vi "DLL Test1.vi"() -> ()   [LabVIEW 2015]
panel:
  out "string":string
  out "Data":string
  out "description":string
  out "VarName":string
  out "initialized array":u8[](array[numeric])
  in  "DLL Path":path
  in  "Load File Path":string="C:\\Users\\Public\\Documents\\National Instruments\\Vision\\Examples\\Images\\Battery\\Image00.jpg"
  in  "Load Template":bool
  in  "coordinate space":bool
  in  "Run":bool
  in  "Enabled/Disabled":bool
  in  "script path":string="C:\\Users\\chenju\\Desktop\\iVision_20160418_Calipter_Coor\\Data\\l"
  in  "stop":bool
  # "<- Run之前要先設定"
  # "<- Run之前要改"
  # "<- Run之前要先設定\n此設定為載入的圖檔"
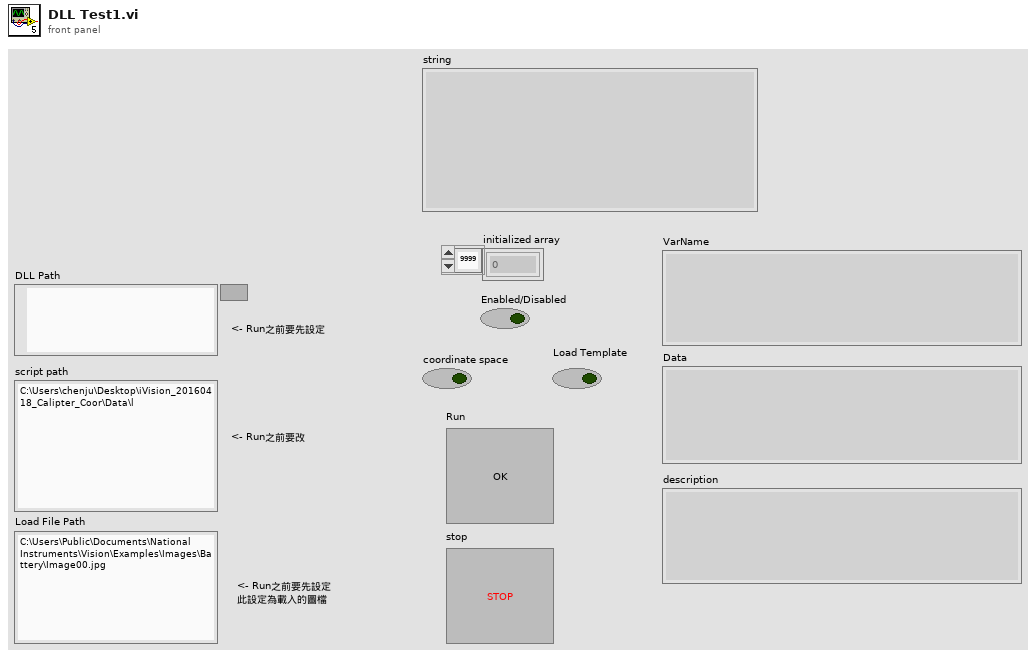
[diagram p1: front panel]
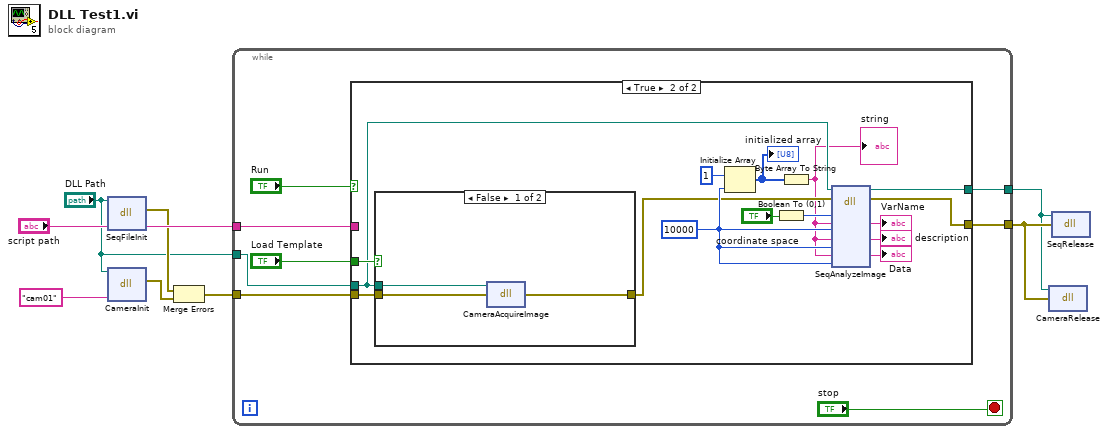
[diagram p0: block diagram]
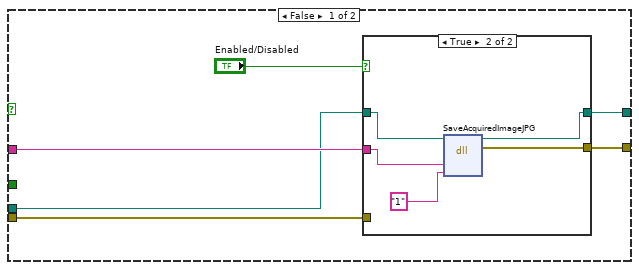
[diagram p2: hidden frame]
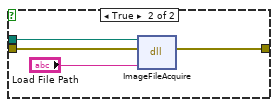
[diagram p4: hidden frame]
diagram:
  n1 = dll-call lib="C:/Users/chenju/Desktop/iVision_20160418_Calipter_Coor/DLL/builds/VisionSeq.dll" fn="SeqFileInit"(path in="DLL Path", "SeqFileInit"="script path") -> (error out=w6:errorcluster, "SeqFileInit"=w7:string)  [unwired: 3 in, 1 out]
  n2 = dll-call lib="C:/Users/chenju/Desktop/iVision_20160418_Calipter_Coor/DLL/builds/VisionSeq.dll" fn="CameraInit"(path in="DLL Path", "CameraInit"="cam01" ("CameraName")) -> (error out=w4:errorcluster)  [unwired: 4 in, 1 out]
  n3 = Merge Errors(w6, w4) -> (w9:errorcluster)
  n4 = while {
    tunnel: w9 -> [w16]
    tunnel: [w15] -> w2
    tunnel: w7 -> [w14]
    tunnel: "DLL Path" -> [w11]
    tunnel: [w10] -> w1
    stop <- "stop" stop-if-true
    n5 = case shown="True" "Run" {
      tunnel: w16 -> [w22 w45]
      tunnel: [w21 w34] -> w15
      tunnel: w14 -> [w20 _]
      tunnel: "Load Template" -> [_ w44]
      tunnel: w11 -> [w18 w33]
      tunnel: [w19 w32] -> w10
      frame False {
        n6 = case shown="True" "Enabled/Disabled" {
          tunnel: w22 -> [w25 _]
          tunnel: [w25 w30] -> w21
          tunnel: w20 -> [_ w27]
          tunnel: [w24 w28] -> w19
          tunnel: w18 -> [w24 w29]
          frame False {
          }
          frame True {
            n7 = dll-call lib="C:/Users/chenju/Desktop/iVision_20160418_Calipter_Coor/DLL/builds/VisionSeq.dll" fn="SaveAcquiredImageJPG"(path in=w29, "Folder Path"=w27, "File Name"="1") -> (path out=w28:path, error out=w30:errorcluster)  [unwired: 5 in]
          }
        }
      }
      frame True {
        w36 = 10000 ("Len")
        n8 = case shown="False" w44 {
          tunnel: w45 -> [w48 w49]
          tunnel: [w47 w50] -> w35
          tunnel: w33 -> [w46 w51]
          frame False {
            n9 = dll-call lib="C:/Users/chenju/Desktop/iVision_20160418_Calipter_Coor/DLL/builds/VisionSeq.dll" fn="CameraAcquireImage"(path in=w46, error in=w48) -> (error out=w47:errorcluster)  [unwired: 2 in, 1 out]
          }
          frame True {
            n10 = dll-call lib="C:/Users/chenju/Desktop/iVision_20160418_Calipter_Coor/DLL/builds/VisionSeq.dll" fn="ImageFileAcquire"(path in=w51, error in=w49, "ImageFileAcquire"="Load File Path") -> (error out=w50:errorcluster)  [unwired: 3 in, 1 out]
          }
        }
        n11 = Initialize Array(1, w36) -> (w41:i32[])
        "initialized array" <- w41
        n12 = Boolean To (0,1)(Boolean="coordinate space") -> (0, 1=w43:i16)
        n13 = Byte Array To String(unsigned byte array=w41) -> (string=w31:string)
        "string" <- w31
        n14 = dll-call lib="C:/Users/chenju/Desktop/iVision_20160418_Calipter_Coor/DLL/builds/VisionSeq.dll" fn="SeqAnalyzeImage"(path in=w33, error in=w35, "coordinate space"=w43, "VarName"=w31, "VarName_len"=w36, "description"=w31, "description_Len"=w36, "Data"=w31, "Data_Len"=w36) -> (path out=w32:path, error out=w34:errorcluster, "VarName"=→"VarName":string, "description"=→"description":string, "Data"=→"Data":string)  [unwired: 6 in]
      }
    }
  }
  n15 = dll-call lib="C:/Users/chenju/Desktop/iVision_20160418_Calipter_Coor/DLL/builds/VisionSeq.dll" fn="CameraRelease"(path in=w1, error in=w2) -> ()  [unwired: 2 in, 2 out]
  n16 = dll-call lib="C:/Users/chenju/Desktop/iVision_20160418_Calipter_Coor/DLL/builds/VisionSeq.dll" fn="SeqRelease"(path in=w1, error in=w2) -> ()  [unwired: 2 in, 2 out]
